vi "Remove Oldest.vi"(8 "error in (no error)":errorcluster, 10 "Min volume free space":i64, 11 "TDMS file path string":path) -> (0 "Error Out":errorcluster)   [LabVIEW 2015]
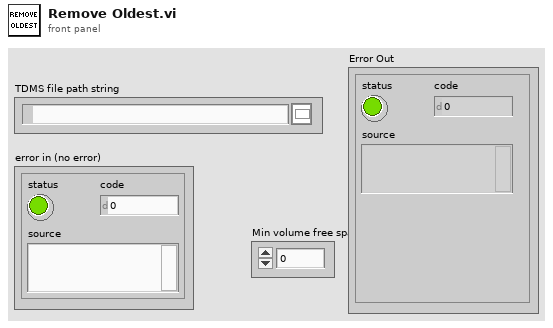
[diagram p1: front panel]
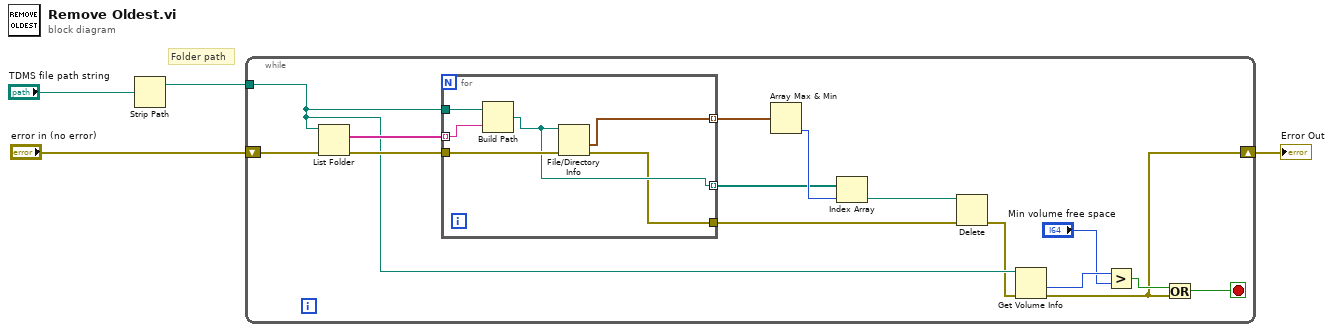
[diagram p0: block diagram]
diagram:
  # "Folder path"
  n1 = Strip Path(path="TDMS file path string") -> (stripped path=w4:path)  [unwired: 1 out]
  n2 = while {
    tunnel: w4 -> [w11]
    shift-right: [w6] -> w1
    shift-left: "error in (no error)" -> [w17]
    stop <- w5 stop-if-true
    n3 = List Folder(path=w11, error in=w17) -> (filenames=w19:string[], error out=w18:errorcluster)  [unwired: 2 in, 2 out]
    n4 = for {
      tunnel: w18 -> [w24]
      tunnel: w19 -> [w22] mode=indexing
      tunnel: w11 -> [w25]
      tunnel: [w23] -> w16 mode=indexing
      tunnel: [w21] -> w14 mode=indexing
      tunnel: [w20] -> w12
      n5 = Build Path(base path=w25, name or relative path=w22) -> (appended path=w21:path)
      n6 = File/Directory Info(path=w21, error in=w24) -> (last mod=w23:timestamp, error out=w20:errorcluster)  [unwired: 5 out]
    }
    n7 = Array Max & Min(array=w16) -> (min index (indices)=w15:i32)  [unwired: 3 out]
    n8 = Index Array(array=w14, index=w15) -> (element=w13:path)
    n9 = Delete(path (use dialog)=w13, error in=w12) -> (error out=w10:errorcluster)  [unwired: 3 in, 2 out]
    n10 = Get Volume Info(8:w10, 11:w11) -> (0:w6:errorcluster, 1:w9:i64)  [unwired: 4 out]
    n11 = Greater?(x=w9, y="Min volume free space") -> (0:w7:bool)
    n12 = Or(x=w7, y=w6) -> (x .or. y?=w5:bool)
  }
  "Error Out" <- w1
